vi "Load and Save Data (Generic Data).vi"(0 "VISA resource name":refnum<visa-resource-name>, 5 "Destination File":string, 7 "Data Block":string, 11 "error in (no error)":errorcluster) -> (4 "VISA resource name out":refnum<visa-resource-name>, 15 "error out":errorcluster)   [LabVIEW 2018, in "Agilent PSG MXG Series.lvlib"]
doc: "Loads data into signal generator memory and saves the data to a file.\n\n<B>Note:</B>\nThis VI is valid on N5171B, N5172B, N5173B, N5181B, N5182B, N5183B, N5161A, N5162A, N5181A, N5182A, N5183A."
uses:
  Agilent PSG MXG Series.lvlib
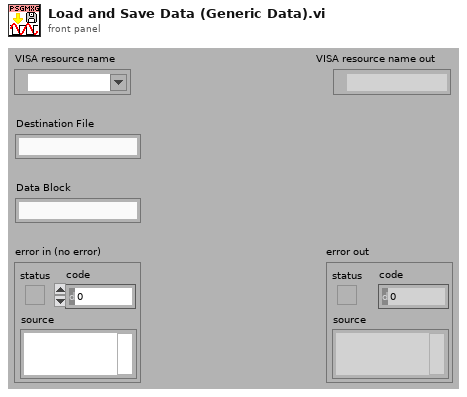
[diagram p1: front panel]
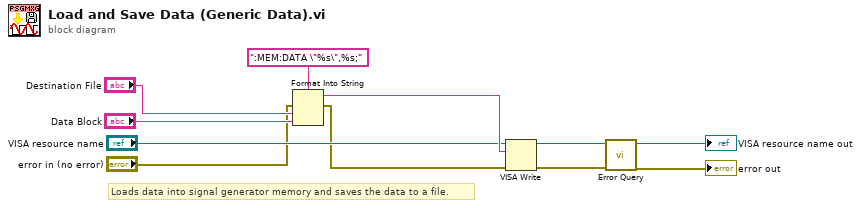
[diagram p0: block diagram]
diagram:
  # "Loads data into signal generator memory and saves the data to a file."
  n1 = Format Into String(format string=":MEM:DATA \"%s\",%s;", error in="error in (no error)", "Destination File", "Data Block") -> (resulting string=w6:string, error out=w1:errorcluster)  [unwired: 1 in]
  n2 = VISA Write(VISA resource name="VISA resource name", write buffer=w6, error in (no error)=w1) -> (VISA resource name out=w11:refnum<visa-resource-name>, error out=w10:errorcluster)  [unwired: 1 out]
  n3 = call "Error Query.vi"("error in (no error)"=w10, "VISA resource name"=w11) -> ("error out"=→"error out":errorcluster, "VISA resource name out"=→"VISA resource name out":refnum<visa-resource-name>)  [unwired: 6 in, 2 out]
